vi "Dequeue Result.vi"(8 "error in (no error)":errorcluster, 9 "timeout in ms (0)":i32, 11 "Mock Report In":refnum<class "Mock Report.lvclass">) -> (0 "error out":errorcluster, 2 "Result":T1={"Name"="", "Description"="", "Status"=enum."Passed", "Result Type"=enum."Test Suite", "Execution Time"=0.0, "Data"={"Expected"=variant, "Actual"=variant, "Delta"=variant}}, 3 "Mock Report Out":refnum<class "Mock Report.lvclass">)   [LabVIEW 2020, in "Mock Report.lvclass"]
uses:
  Mock Report.lvclass
  source/Core/Result/Result.ctl
  source/Core/Result/Status.ctl
  source/Core/Result/Type.ctl
  Mock Report.lvclass/Mock Report.ctl
  source/Core/Result/Result.lvlib
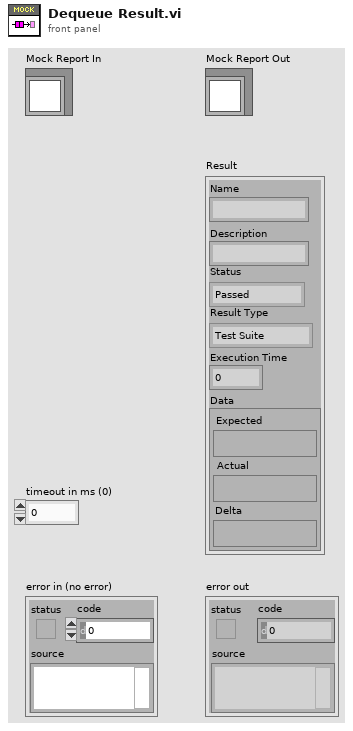
[diagram p1: front panel]
types:
  T1 = typedef "Result.lvlib/Result.ctl" = cluster{"Name":string, "Description":string, "Status":T2, "Result Type":T3, "Execution Time":dbl, "Data":cluster{"Expected":variant, "Actual":variant, "Delta":variant}}
  T2 = typedef "Result.lvlib/Status.ctl" = enum16{"", "Passed", "Failed", "Error", "Skipped", "Setup Error", "Broken", "Teardown Error"}
  T3 = typedef "Result.lvlib/Type.ctl" = enum16{"Test Case", "Test Suite", "Test Run", "Pass", "Fail", "Skip", "Pass if", "Fail if", "Pass if Error", "Fail if Error", "Pass if Equal", "Fail if Equal"}
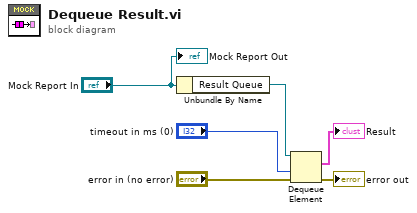
[diagram p0: block diagram]
diagram:
  n1 = Unbundle By Name("Mock Report In") -> ("Result Queue"=w2:refnum<queue>)
  n2 = Dequeue Element(queue=w2, timeout in ms (-1)="timeout in ms (0)", error in (no error)="error in (no error)") -> (element=→"Result":T1, error out=→"error out":errorcluster)  [unwired: 2 out]
  "Mock Report Out" <- "Mock Report In"
